vi "OutbitsCleanUpAfterScan.vi"   [LabVIEW 2014]
panel:
  # "sets alle outbits to false\nand erases all commands from memory"
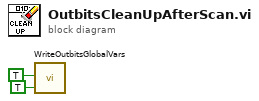
[diagram p0: block diagram]
diagram:
  n1 = call "WriteOutbitsGlobalVars.vi"("write_OutBitStopListening"=TRUE, "OutBitStopListening"=TRUE) -> ()  [unwired: 17 in, 1 out]
